vi "CloseTrig.vi"(8 "error in (no error)":errorcluster, 10 "ClkName":string, 11 "NiPxi6683H in":refnum<class "NiPxi6683H.lvclass">) -> (0 "error out":errorcluster, 3 "NiPxi6683H out":refnum<class "NiPxi6683H.lvclass">)   [LabVIEW 2014, in "SyncPlugins.lvlib" / "NiPxi6683H.lvclass"]
uses:
  NiPxi6683H.lvclass
  NiPxi6683H.lvclass/NiPxi6683H.ctl
  NiPxi6682/NiPxi6682.lvclass/NiPxi6682.ctl
  NiPxi6682/Accessors/Read NiSyncHandle.vi
  NiPxi6682/Accessors/Write NiSyncHandle.vi
  Accessors/Write Triggers.vi
  Accessors/Read Triggers.vi
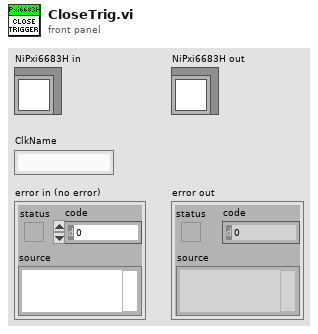
[diagram p1: front panel]
types:
  T1 = typedef "SyncPlugins.lvlib/PXI_MultiTrig.lvclass/clTrigger.ctl" = cluster{"Name":string, "DestTerm":string, "SrcTerm":string, "SyncClk":string, "Edge":i32, "Invert?":i32, "Initiated":bool, "Type":string, "TrigTime":bool}
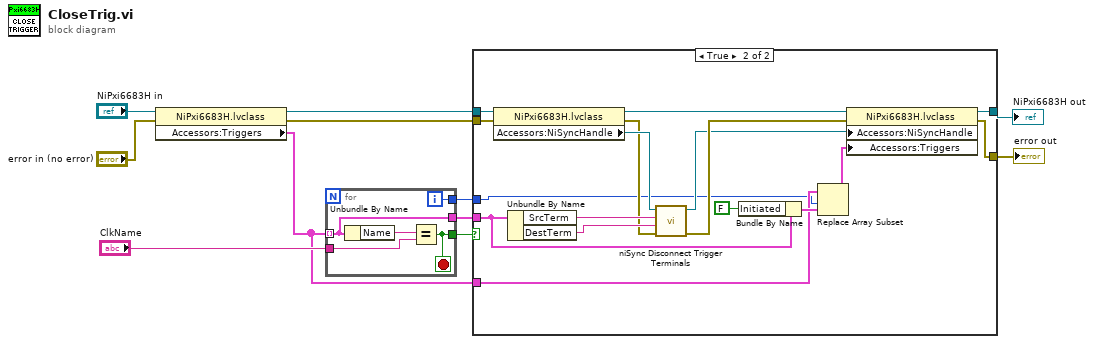
[diagram p0: block diagram]
diagram:
  n1 = property class="NiPxi6683H.lvclass"(reference="NiPxi6683H in", error in="error in (no error)") -> (reference out=w5:refnum<class "NiPxi6683H.lvclass">, error out=w4:errorcluster, "Accessors:Triggers"=w3:T1[])
  n2 = for {
    tunnel: w3 -> [w13] mode=indexing
    tunnel: "ClkName" -> [w15]
    tunnel: [w14] -> w8
    tunnel: [w13] -> w7
    tunnel: [w12] -> w6
    i -> [w12]
    stop <- w14 stop-if-true
    n3 = Unbundle By Name(w13) -> ("Name"=w16:string)
    n4 = Equal?(x=w16, y=w15) -> (x = y?=w14:bool)
  }
  n5 = case shown="True" w8 {
    tunnel: w7 -> [_ w29]
    tunnel: w6 -> [_ w22]
    tunnel: w5 -> [w18 w35]
    tunnel: w4 -> [w17 w34]
    tunnel: w3 -> [_ w23]
    tunnel: [w18 w20] -> w2
    tunnel: [w17 w19] -> w1
    frame False {
    }
    frame True {
      n6 = property class="NiPxi6683H.lvclass"(reference=w35, error in=w34) -> (reference out=w27:refnum<class "NiPxi6683H.lvclass">, error out=w30:errorcluster, "Accessors:NiSyncHandle"=w31:refnum<k15>)
      n7 = Unbundle By Name(w29) -> ("SrcTerm"=w33:string, "DestTerm"=w32:string)
      n8 = call <instrlib>:"niSync Disconnect Trigger Terminals.vi"("error in (no error)"=w30, "destination terminal"=w32, "source terminal"=w33, "instrument handle"=w31) -> ("error out"=w26:errorcluster, "instrument handle out"=w25:refnum<k15>)  [unwired: 6 in]
      n9 = Bundle By Name(cluster=w29, "Initiated"=FALSE) -> (w24:T1)
      n10 = Replace Array Subset(array=w23, new element=w24, index=w22) -> (w21:T1[])
      n11 = property class="NiPxi6683H.lvclass"(reference=w27, error in=w26, "Accessors:NiSyncHandle"=w25, "Accessors:Triggers"=w21) -> (reference out=w20:refnum<class "NiPxi6683H.lvclass">, error out=w19:errorcluster)
    }
  }
  "error out" <- w1
  "NiPxi6683H out" <- w2
